vi "Edge Trigger.vi"(1 "Signal":bool) -> (0 "Trigger?":bool)   [LabVIEW 2013]
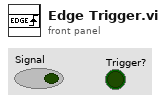
[diagram p1: front panel]
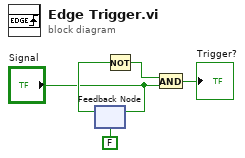
[diagram p0: block diagram]
diagram:
  n1 = feedback #1(FALSE ("Signal")) -> (w4:bool)
  n2 = feedback-in #1("Signal") -> ()
  n3 = Not(x=w4) -> (.not. x?=w3:bool)
  n4 = And(x=w3, y="Signal") -> (x .and. y?=→"Trigger?":bool)
